vi "HDF5_Write_Weather_Record.vi"(8 "error in":errorcluster, 10 "WeatherData":T1, 11 "WeathRefs":T3 {"WindDirSTD_dset" format="%.0x"; "WindGusts_dset" format="%.0x"; "RainFall_dset" format="%.0x"; "RainRate_dset" format="%.0x"; "Pressure_dset" format="%.0x"; "Humidity_dset" format="%.0x"; "Temp_dset" format="%.0x"; "WindDir_dset" format="%.0x"; "WindSpd_dset" format="%.0x"; "TimeStamp_dset" format="%.0x"; "Group_ref" format="%.0x"; "TimeString_dset" format="%.0x"}) -> (0 "error out":errorcluster)   [LabVIEW 2018]
doc: "Write a single Tone<x> record with timestamp:\nTone1\n Beac - cluster\n BeacZoom - 1024 element Double array (waveform) \n Cal - cluster\n CalZoom - 1024 element Double array (waveform)"
uses:
  Controls/Clusts/WeatherRefs.ctl
  <vilib>/addons/h5labview2/base/hid_t.ctl
  Controls/Clusts/WeatherDataClust.ctl
  Controls/Clusts/ValidityWeatherClust.ctl
  lib_path_mod_20200519.vi
  <vilib>/addons/h5labview2/base/H5Equery.vi
  <vilib>/addons/h5labview2/dataset/H5Dwrite.llb/H5Dwrite.xnode
  <vilib>/addons/h5labview2/dataset/H5D.lvlib
  <vilib>/addons/h5labview2/space/H5S.lvlib
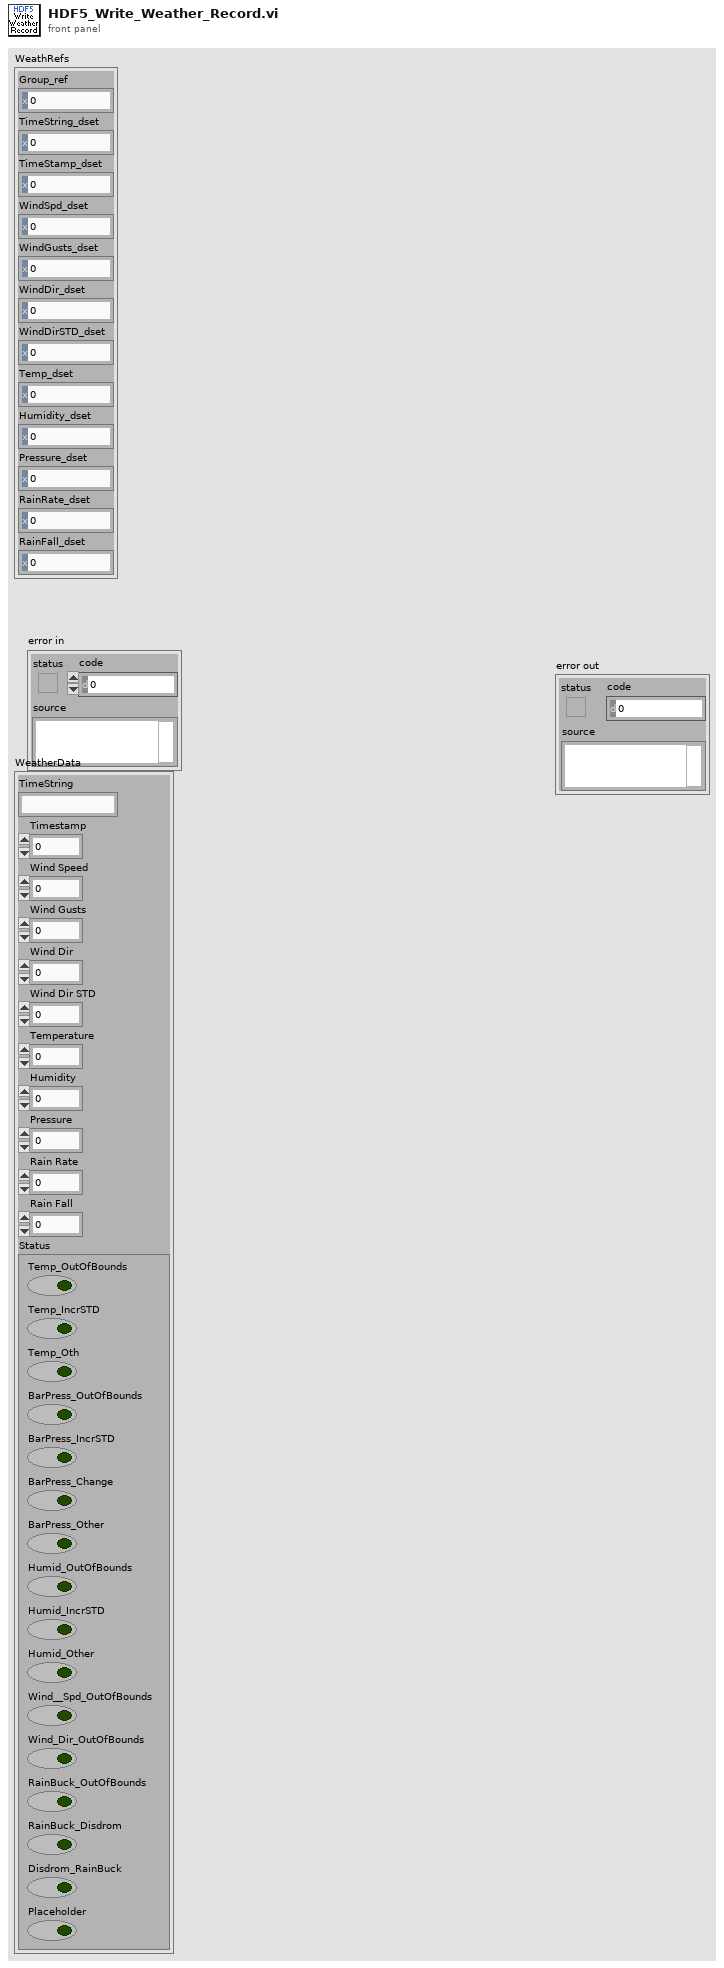
[diagram p1: front panel]
types:
  T1 = typedef "WeatherDataClust.ctl" = cluster{"TimeString":string, "Timestamp":dbl, "Wind Speed":sgl, "Wind Gusts":sgl, "Wind Dir":sgl, "Wind Dir STD":sgl, "Temperature":sgl, "Humidity":sgl, "Pressure":sgl, "Rain Rate":i16, "Rain Fall":sgl, "Status":T2}
  T2 = typedef "ValidityWeatherClust.ctl" = cluster{"Temp_OutOfBounds":bool, "Temp_IncrSTD":bool, "Temp_Oth":bool, "BarPress_OutOfBounds":bool, "BarPress_IncrSTD":bool, "BarPress_Change":bool, "BarPress_Other":bool, "Humid_OutOfBounds":bool, "Humid_IncrSTD":bool, "Humid_Other":bool, "Wind__Spd_OutOfBounds":bool, "Wind_Dir_OutOfBounds":bool, "RainBuck_OutOfBounds":bool, "RainBuck_Disdrom":bool, "Disdrom_RainBuck":bool, "Placeholder":bool}
  T3 = typedef "WeatherRefs.ctl" = cluster{"Group_ref":T4, "TimeString_dset":T4, "TimeStamp_dset ":T4, "WindSpd_dset":T4, "WindGusts_dset":T4, "WindDir_dset":T4, "WindDirSTD_dset":T4, "Temp_dset":T4, "Humidity_dset":T4, "Pressure_dset":T4, "RainRate_dset":T4, "RainFall_dset":T4}
  T4 = typedef "hid_t.ctl" = i32
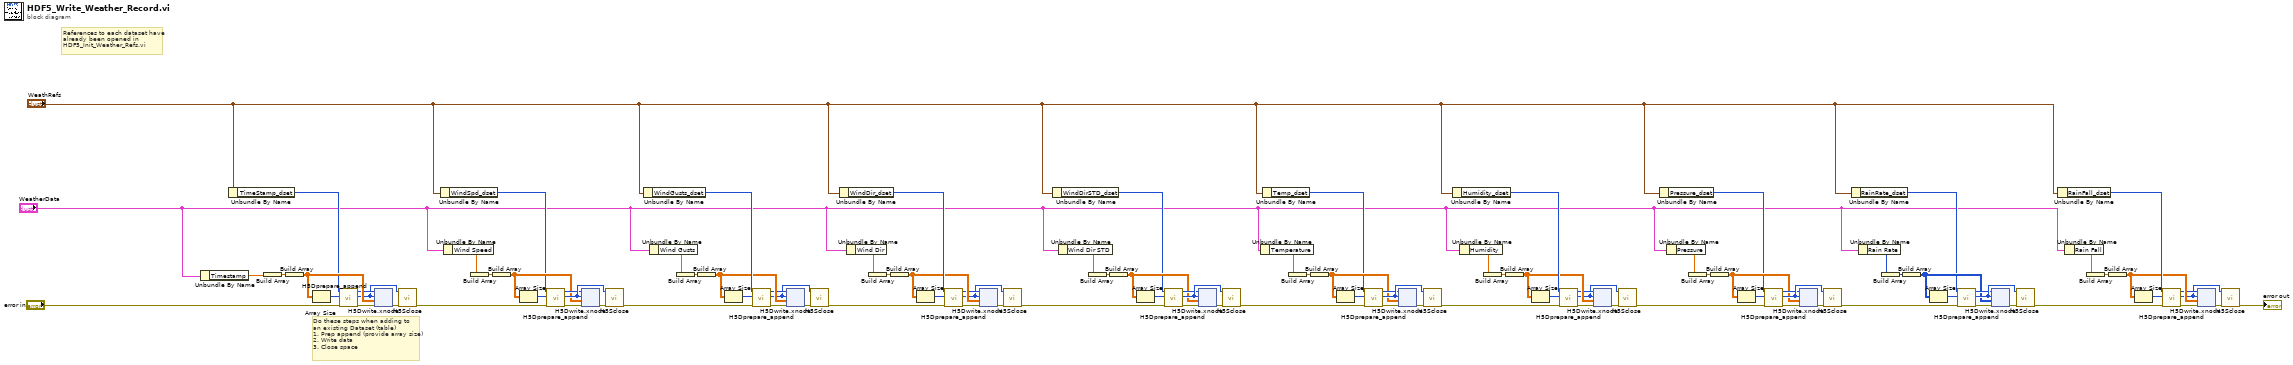
[diagram p0: block diagram]
diagram:
  # "References to each dataset have \nalready been opened in \nHDF5_Init_Weather_Refs.vi"
  # "Do these steps when adding to \nan existing Dataset (table)\n1. Prep append (provide array size)\n2. Write data\n3. Close space"
  n1 = Unbundle By Name("WeatherData") -> ("Timestamp"=w1:dbl)
  n2 = Unbundle By Name("WeathRefs") -> ("TimeStamp_dset"=w89:T4)
  n3 = Build Array(w1) -> (w101:dbl[])
  n4 = Build Array(w101) -> (w102:dbl[][])
  n5 = Array Size(array=w102) -> (size(s)=w103:i32[])
  n6 = call <vilib>:"H5Dprepare_append.vi"("error in (no error)"="error in", "append dims"=w103, "dset in"=w89) -> ("error out"=w97:errorcluster, "space out"=w99:T4, "dset out"=w100:T4)  [unwired: 5 in, 1 out]
  n7 = xnode "H5Dwrite.xnode"("error in (no error)"=w97, "data"=w102, "file space"=w99, "ref in"=w100) -> ("error out"=w98:errorcluster)  [unwired: 3 in, 2 out]
  n8 = call <vilib>:"H5Sclose.vi"("error in (no error)"=w98, "space in"=w99) -> ("error out"=w23:errorcluster)  [unwired: 9 in]
  n9 = Unbundle By Name("WeathRefs") -> ("WindSpd_dset"=w87:T4)
  n10 = Unbundle By Name("WeatherData") -> ("Wind Speed"=w88:sgl)
  n11 = Build Array(w88) -> (w92:sgl[])
  n12 = Build Array(w92) -> (w91:sgl[][])
  n13 = Array Size(array=w91) -> (size(s)=w90:i32[])
  n14 = call <vilib>:"H5Dprepare_append.vi"("error in (no error)"=w23, "append dims"=w90, "dset in"=w87) -> ("error out"=w96:errorcluster, "space out"=w94:T4, "dset out"=w93:T4)  [unwired: 5 in, 1 out]
  n15 = xnode "H5Dwrite.xnode"("error in (no error)"=w96, "data"=w91, "file space"=w94, "ref in"=w93) -> ("error out"=w95:errorcluster)  [unwired: 3 in, 2 out]
  n16 = call <vilib>:"H5Sclose.vi"("error in (no error)"=w95, "space in"=w94) -> ("error out"=w22:errorcluster)  [unwired: 9 in]
  n17 = Unbundle By Name("WeathRefs") -> ("WindGusts_dset"=w86:T4)
  n18 = Unbundle By Name("WeatherData") -> ("Wind Gusts"=w85:sgl)
  n19 = Build Array(w85) -> (w82:sgl[])
  n20 = Build Array(w82) -> (w83:sgl[][])
  n21 = Array Size(array=w83) -> (size(s)=w84:i32[])
  n22 = call <vilib>:"H5Dprepare_append.vi"("error in (no error)"=w22, "append dims"=w84, "dset in"=w86) -> ("error out"=w78:errorcluster, "space out"=w80:T4, "dset out"=w81:T4)  [unwired: 5 in, 1 out]
  n23 = xnode "H5Dwrite.xnode"("error in (no error)"=w78, "data"=w83, "file space"=w80, "ref in"=w81) -> ("error out"=w79:errorcluster)  [unwired: 3 in, 2 out]
  n24 = call <vilib>:"H5Sclose.vi"("error in (no error)"=w79, "space in"=w80) -> ("error out"=w21:errorcluster)  [unwired: 9 in]
  n25 = Unbundle By Name("WeathRefs") -> ("WindDir_dset"=w68:T4)
  n26 = Unbundle By Name("WeatherData") -> ("Wind Dir"=w67:sgl)
  n27 = Build Array(w67) -> (w64:sgl[])
  n28 = Build Array(w64) -> (w65:sgl[][])
  n29 = Array Size(array=w65) -> (size(s)=w66:i32[])
  n30 = call <vilib>:"H5Dprepare_append.vi"("error in (no error)"=w21, "append dims"=w66, "dset in"=w68) -> ("error out"=w60:errorcluster, "space out"=w62:T4, "dset out"=w63:T4)  [unwired: 5 in, 1 out]
  n31 = xnode "H5Dwrite.xnode"("error in (no error)"=w60, "data"=w65, "file space"=w62, "ref in"=w63) -> ("error out"=w61:errorcluster)  [unwired: 3 in, 2 out]
  n32 = call <vilib>:"H5Sclose.vi"("error in (no error)"=w61, "space in"=w62) -> ("error out"=w6:errorcluster)  [unwired: 9 in]
  n33 = Unbundle By Name("WeathRefs") -> ("WindDirSTD_dset"=w7:T4)
  n34 = Unbundle By Name("WeatherData") -> ("Wind Dir STD"=w8:sgl)
  n35 = Build Array(w8) -> (w11:sgl[])
  n36 = Build Array(w11) -> (w10:sgl[][])
  n37 = Array Size(array=w10) -> (size(s)=w9:i32[])
  n38 = call <vilib>:"H5Dprepare_append.vi"("error in (no error)"=w6, "append dims"=w9, "dset in"=w7) -> ("error out"=w15:errorcluster, "space out"=w13:T4, "dset out"=w12:T4)  [unwired: 5 in, 1 out]
  n39 = xnode "H5Dwrite.xnode"("error in (no error)"=w15, "data"=w10, "file space"=w13, "ref in"=w12) -> ("error out"=w14:errorcluster)  [unwired: 3 in, 2 out]
  n40 = call <vilib>:"H5Sclose.vi"("error in (no error)"=w14, "space in"=w13) -> ("error out"=w5:errorcluster)  [unwired: 9 in]
  n41 = Unbundle By Name("WeatherData") -> ("Temperature"=w70:sgl)
  n42 = Unbundle By Name("WeathRefs") -> ("Temp_dset"=w69:T4)
  n43 = Build Array(w70) -> (w73:sgl[])
  n44 = Build Array(w73) -> (w72:sgl[][])
  n45 = Array Size(array=w72) -> (size(s)=w71:i32[])
  n46 = call <vilib>:"H5Dprepare_append.vi"("error in (no error)"=w5, "append dims"=w71, "dset in"=w69) -> ("error out"=w77:errorcluster, "space out"=w75:T4, "dset out"=w74:T4)  [unwired: 5 in, 1 out]
  n47 = xnode "H5Dwrite.xnode"("error in (no error)"=w77, "data"=w72, "file space"=w75, "ref in"=w74) -> ("error out"=w76:errorcluster)  [unwired: 3 in, 2 out]
  n48 = call <vilib>:"H5Sclose.vi"("error in (no error)"=w76, "space in"=w75) -> ("error out"=w20:errorcluster)  [unwired: 9 in]
  n49 = Unbundle By Name("WeathRefs") -> ("Humidity_dset"=w32:T4)
  n50 = Unbundle By Name("WeatherData") -> ("Humidity"=w31:sgl)
  n51 = Build Array(w31) -> (w28:sgl[])
  n52 = Build Array(w28) -> (w29:sgl[][])
  n53 = Array Size(array=w29) -> (size(s)=w30:i32[])
  n54 = call <vilib>:"H5Dprepare_append.vi"("error in (no error)"=w20, "append dims"=w30, "dset in"=w32) -> ("error out"=w24:errorcluster, "space out"=w26:T4, "dset out"=w27:T4)  [unwired: 5 in, 1 out]
  n55 = xnode "H5Dwrite.xnode"("error in (no error)"=w24, "data"=w29, "file space"=w26, "ref in"=w27) -> ("error out"=w25:errorcluster)  [unwired: 3 in, 2 out]
  n56 = call <vilib>:"H5Sclose.vi"("error in (no error)"=w25, "space in"=w26) -> ("error out"=w19:errorcluster)  [unwired: 9 in]
  n57 = Unbundle By Name("WeathRefs") -> ("Pressure_dset"=w33:T4)
  n58 = Unbundle By Name("WeatherData") -> ("Pressure"=w34:sgl)
  n59 = Build Array(w34) -> (w37:sgl[])
  n60 = Build Array(w37) -> (w36:sgl[][])
  n61 = Array Size(array=w36) -> (size(s)=w35:i32[])
  n62 = call <vilib>:"H5Dprepare_append.vi"("error in (no error)"=w19, "append dims"=w35, "dset in"=w33) -> ("error out"=w41:errorcluster, "space out"=w39:T4, "dset out"=w38:T4)  [unwired: 5 in, 1 out]
  n63 = xnode "H5Dwrite.xnode"("error in (no error)"=w41, "data"=w36, "file space"=w39, "ref in"=w38) -> ("error out"=w40:errorcluster)  [unwired: 3 in, 2 out]
  n64 = call <vilib>:"H5Sclose.vi"("error in (no error)"=w40, "space in"=w39) -> ("error out"=w18:errorcluster)  [unwired: 9 in]
  n65 = Unbundle By Name("WeathRefs") -> ("RainRate_dset"=w51:T4)
  n66 = Unbundle By Name("WeatherData") -> ("Rain Rate"=w52:i16)
  n67 = Build Array(w52) -> (w55:i16[])
  n68 = Build Array(w55) -> (w54:i16[][])
  n69 = Array Size(array=w54) -> (size(s)=w53:i32[])
  n70 = call <vilib>:"H5Dprepare_append.vi"("error in (no error)"=w18, "append dims"=w53, "dset in"=w51) -> ("error out"=w59:errorcluster, "space out"=w57:T4, "dset out"=w56:T4)  [unwired: 5 in, 1 out]
  n71 = xnode "H5Dwrite.xnode"("error in (no error)"=w59, "data"=w54, "file space"=w57, "ref in"=w56) -> ("error out"=w58:errorcluster)  [unwired: 3 in, 2 out]
  n72 = call <vilib>:"H5Sclose.vi"("error in (no error)"=w58, "space in"=w57) -> ("error out"=w17:errorcluster)  [unwired: 9 in]
  n73 = Unbundle By Name("WeathRefs") -> ("RainFall_dset"=w50:T4)
  n74 = Unbundle By Name("WeatherData") -> ("Rain Fall"=w49:sgl)
  n75 = Build Array(w49) -> (w46:sgl[])
  n76 = Build Array(w46) -> (w47:sgl[][])
  n77 = Array Size(array=w47) -> (size(s)=w48:i32[])
  n78 = call <vilib>:"H5Dprepare_append.vi"("error in (no error)"=w17, "append dims"=w48, "dset in"=w50) -> ("error out"=w42:errorcluster, "space out"=w44:T4, "dset out"=w45:T4)  [unwired: 5 in, 1 out]
  n79 = xnode "H5Dwrite.xnode"("error in (no error)"=w42, "data"=w47, "file space"=w44, "ref in"=w45) -> ("error out"=w43:errorcluster)  [unwired: 3 in, 2 out]
  n80 = call <vilib>:"H5Sclose.vi"("error in (no error)"=w43, "space in"=w44) -> ("error out"=→"error out":errorcluster)  [unwired: 9 in]
